vi "UI Loop Error and Que Setup.vi"(8 "error in (no error)":errorcluster, 11 "Receive Loop":refnum<user-event>) -> (0 "error out":errorcluster, 1 "UI Loop Event Registration":refnum<event-registration>, 3 "GEA Display Queue":refnum<queue>, 5 "ERD Queue Loop":refnum<queue>)   [LabVIEW 2023]
uses:
  Common/type defs/ERD_Data_Loop_Control.ctl
  Common/type defs/ERD_Loop_States.ctl
  Common/GExplorer Support/typedefs/GExplorer_Data_Cluster.ctl
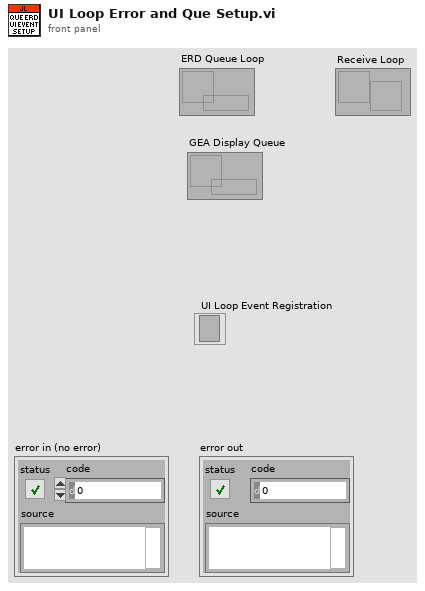
[diagram p1: front panel]
types:
  T1 = typedef "GExplorer_Data_Cluster.ctl" = cluster{"Data":variant, "State":enum16{"Add to Log", "Clear", "Shutdown"}}
  T2 = typedef "ERD_Data_Loop_Control.ctl" = cluster{"Data":variant, "State":T3}
  T3 = typedef "ERD_Loop_States.ctl" = enum16{"Init", "Build ERD Read List", "Read ERDs", "Get Version", "ERD´s User show", "Update UI", "Graph", "Read Faults", "Log Data", "Pause", "Shutdown"}
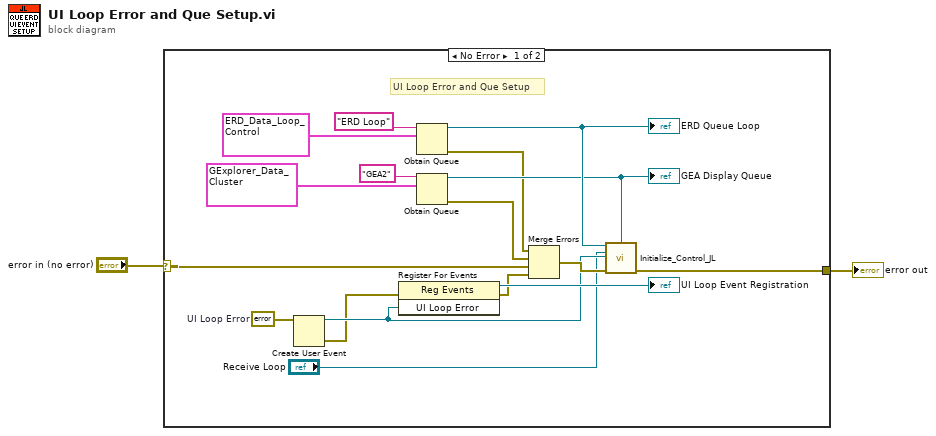
[diagram p0: block diagram]
diagram:
  n1 = case shown="No Error" "error in (no error)" {
    selector: "error in (no error)" -> [w4 w20]
    tunnel: [w19 w20] -> w2
    frame No Error {
      w7 = errorcluster {"status"=FALSE, "code"=0, "source"=""}  # UI Loop Error
      # "UI Loop Error and Que Setup"
      n2 = Create User Event(user event datatype=w7) -> (user event=w11:refnum<user-event>, error out=w8:errorcluster)  [unwired: 1 in]
      n3 = register-events(error in=w8, w11) -> (reference out=→"UI Loop Event Registration":refnum<event-registration>, error out=w3:errorcluster)  [unwired: 1 in]
      n4 = Obtain Queue(name (unnamed)="ERD Loop", element data type=T2 {"Data"=variant, "State"=enum."Read ERDs"} ("Data")) -> (queue out=w17:refnum<queue>, error out=w15:errorcluster)  [unwired: 3 in, 1 out]
      "ERD Queue Loop" <- w17
      n5 = Obtain Queue(name (unnamed)="GEA2", element data type=T1 {"Data"=variant, "State"=enum."Add to Log"} ("Data")) -> (queue out=w16:refnum<queue>, error out=w13:errorcluster)  [unwired: 3 in, 1 out]
      "GEA Display Queue" <- w16
      n6 = Merge Errors(w15, w13, w4, w3) -> (w14:errorcluster)
      n7 = call "Initialize_Control_JL.vi"("ERD Loop"=w17, "GEA2"=w16, "Receive Loop"="Receive Loop", "UI Loop Error"=w11, "Error In"=w14) -> ("Error Out"=w19:errorcluster)  [unwired: 10 in]
    }
    frame Error {
    }
  }
  "error out" <- w2
